vi "SQL_OUT Stack  Insert Cmd.vi"(11 "parameter buffer":T1) -> (1 "结果":string, 2 "净重":string, 3 "连接的字符串":string)   [LabVIEW 2015]
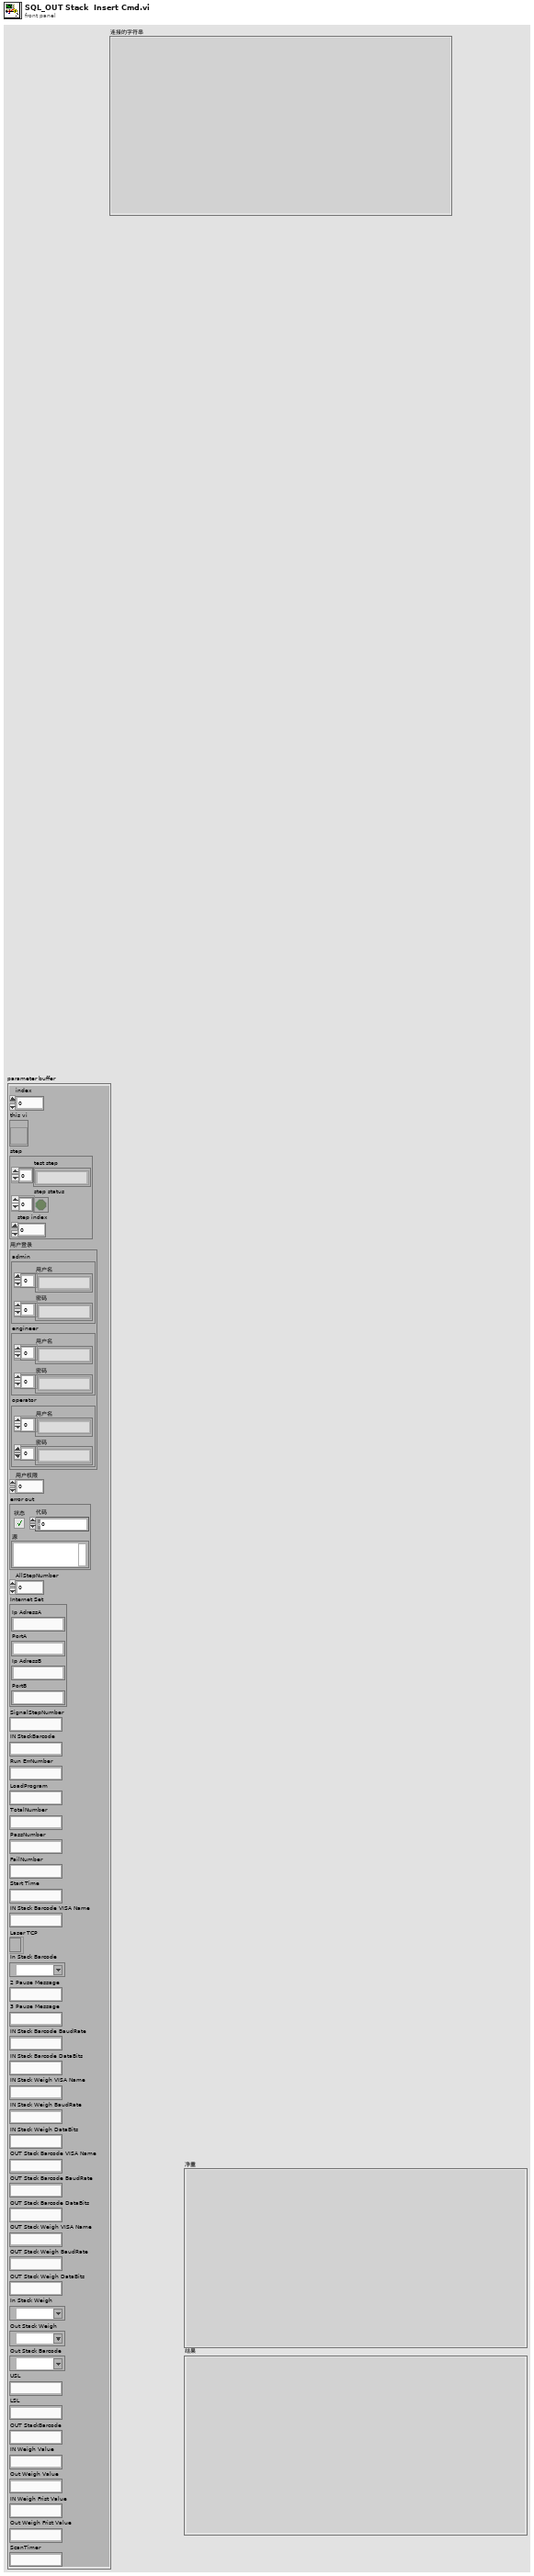
[diagram p1: front panel]
types:
  T1 = cluster{"index":i32, "this vi":refnum<vi>, "step":cluster{"test step":string[], "step status":bool[], "step index":i32}, "用户登录":cluster{"admin":cluster{"用户名":string[], "密码":string[]}, "engineer":cluster{"用户名":string[], "密码":string[]}, "operator":cluster{"用户名":string[], "密码":string[]}}, "用户权限":i32, "error out":errorcluster, "AllStepNumber":i32, "Internet Set":cluster{"Ip AdressA":string, "PortA":string, "Ip AdressB":string, "PortB":string}, "SignalStepNumber":string, "IN StackBarcode":string, "Run ErrNumber":string, "LoadProgram":string, "TotalNumber":string, "PassNumber":string, "FailNumber":string, "Start Time":string, "IN Stack Barcode VISA Name":string, "Laser TCP":refnum<k5>, "In Stack Barcode":refnum<visa-resource-name>, "2 Pause Message":string, "3 Pause Message":string, "IN Stack Barcode BaudRate":string, "IN Stack Barcode DataBits":string, "IN Stack Weigh VISA Name":string, "IN Stack Weigh BaudRate":string, "IN Stack Weigh DataBits":string, "OUT Stack Barcode VISA Name":string, "OUT Stack Barcode BaudRate":string, "OUT Stack Barcode DataBits":string, "OUT Stack Weigh VISA Name":string, "OUT Stack Weigh BaudRate":string, "OUT Stack Weigh DataBits":string, "In Stack Weigh":refnum<visa-resource-name>, "Out Stack Weigh":refnum<visa-resource-name>, "Out Stack Barcode":refnum<visa-resource-name>, "USL":string, "LSL":string, "OUT StackBarcode":string, "IN Weigh Value":string, "Out Weigh Value":string, "IN Weigh Frist Value":string, "Out Weigh Frist Value":string, "ScanTimer":string}
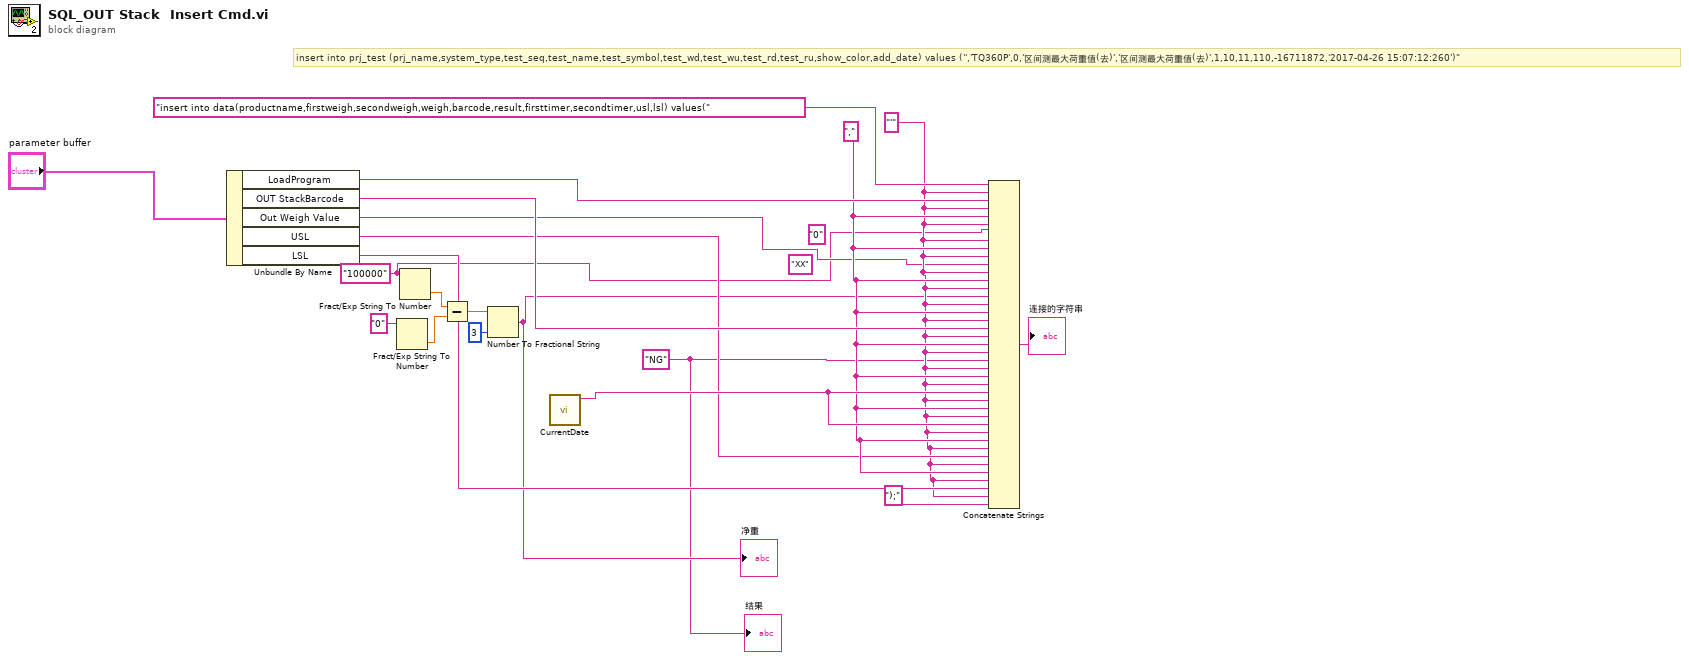
[diagram p0: block diagram]
diagram:
  w2 = "NG" ("字符串")
  (unwired) "0" ("字符串")
  w1 = "100000" ("字符串")
  (unwired) "XX" ("字符串")
  w13 = ","
  w5 = "'"
  # "insert into prj_test (prj_name,system_type,test_seq,test_name,test_symbol,test_wd,test_wu,test_rd,test_ru,show_color,add_date) values ('','TQ360P',0,'区间测最大荷重值(去)','区间测最大荷重值(去)',1,10,11,110,-16711872,'2017-04-26 15:07:12:260')\""
  n1 = Unbundle By Name("parameter buffer") -> ("LoadProgram"=w19:string, "OUT StackBarcode"=w18:string, "Out Weigh Value"=w4:string, "USL"=w12:string, "LSL"=w16:string)
  n2 = Fract/Exp String To Number(string="0" ("字符串")) -> (number=w10:dbl)  [unwired: 3 in, 1 out]
  n3 = Fract/Exp String To Number(string=w1) -> (number=w11:dbl)  [unwired: 3 in, 1 out]
  n4 = Subtract(x=w11, y=w10) -> (x-y=w9:dbl)
  n5 = Number To Fractional String(number=w9, precision (6)=i16 3 ("精度(6)")) -> (F-format string=w3:string)  [unwired: 2 in]
  "净重" <- w3
  n6 = call "CurrentDate.vi"() -> ("当前日期时间"=w17:string)  [unwired: 11 in]
  n7 = Concatenate Strings("insert into data(productname,firstweigh,secondweigh,weigh,barcode,result,firsttimer,secondtimer,usl,lsl) values(" ("字符串"), w5, w19, w5, w13, w5, w1, w5, w13, w5, w4, w5, w13, w5, w3, w5, w13, w5, w18, w5, w13, w5, w2, w5, w13, w5, w17, w5, w13, w5, w17, w5, w13, w5, w12, w5, w13, w5, w16, w5, ");") -> (→"连接的字符串":string)
  "结果" <- w2
